vi "Sub-command.vi"(0 "垂直-降":bool, 1 "垂直-升":bool, 5 "水平-縮":bool, 7 "水平-伸":bool, 9 "停止動作":bool, 12 "開始":bool, 13 "暫停":bool) -> (2 "水平-縮_輸出":bool, 3 "水平-伸_輸出":bool, 4 "垂直-降_輸出":bool, 6 "垂直-升_輸出":bool, 8 "開始_輸出":bool, 10 "停止動作_輸出":bool, 14 "暫停_輸出":bool)   [LabVIEW 2017]
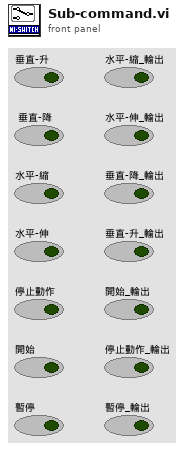
[diagram p1: front panel]
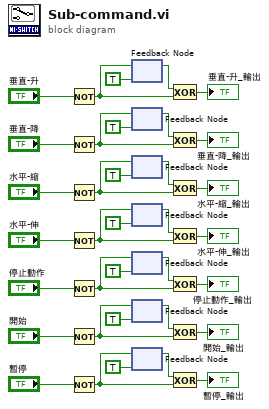
[diagram p0: block diagram]
diagram:
  n1 = Not(x="垂直-升") -> (.not. x?=w17:bool)
  n2 = Not(x="垂直-降") -> (.not. x?=w20:bool)
  n3 = Not(x="水平-縮") -> (.not. x?=w23:bool)
  n4 = Not(x="水平-伸") -> (.not. x?=w26:bool)
  n5 = Not(x="停止動作") -> (.not. x?=w29:bool)
  n6 = Not(x="開始") -> (.not. x?=w32:bool)
  n7 = Not(x="暫停") -> (.not. x?=w35:bool)
  n8 = feedback #1(TRUE ("DI Value")) -> (w16:bool)
  n9 = feedback-in #1(w17) -> ()
  n10 = feedback #2(TRUE ("DI Value")) -> (w19:bool)
  n11 = feedback-in #2(w20) -> ()
  n12 = feedback #3(TRUE ("DI Value")) -> (w22:bool)
  n13 = feedback-in #3(w23) -> ()
  n14 = feedback #4(TRUE ("DI Value")) -> (w25:bool)
  n15 = feedback-in #4(w26) -> ()
  n16 = feedback #5(TRUE ("DI Value")) -> (w28:bool)
  n17 = feedback-in #5(w29) -> ()
  n18 = feedback #6(TRUE ("DI Value")) -> (w31:bool)
  n19 = feedback-in #6(w32) -> ()
  n20 = feedback #7(TRUE ("DI Value")) -> (w34:bool)
  n21 = feedback-in #7(w35) -> ()
  n22 = Exclusive Or(1:w17, 2:w16) -> (0:→"垂直-升_輸出":bool)
  n23 = Exclusive Or(1:w20, 2:w19) -> (0:→"垂直-降_輸出":bool)
  n24 = Exclusive Or(1:w23, 2:w22) -> (0:→"水平-縮_輸出":bool)
  n25 = Exclusive Or(1:w26, 2:w25) -> (0:→"水平-伸_輸出":bool)
  n26 = Exclusive Or(1:w29, 2:w28) -> (0:→"停止動作_輸出":bool)
  n27 = Exclusive Or(1:w32, 2:w31) -> (0:→"開始_輸出":bool)
  n28 = Exclusive Or(1:w35, 2:w34) -> (0:→"暫停_輸出":bool)
